vi "Leap Screen Tap Gesture.vi"() -> ()   [LabVIEW 2011, in "LVH-Leap.lvlib"]
uses:
  vi.lib/LabVIEW Hacker/Leap/LVH-Leap.lvlib
  vi.lib/LabVIEW Hacker/Leap/Public/Gestures/Screen Tap/Instance VIs/Read 1 Screen Tap Position.vi
panel:
  out "Last Screen Tap Position":cluster{"X":sgl, "Y":sgl, "Z":sgl}
  out "X Y Screen Tap Position":cluster{"X":sgl, "Z":sgl}[](graph)
  in  "Stop Button":bool
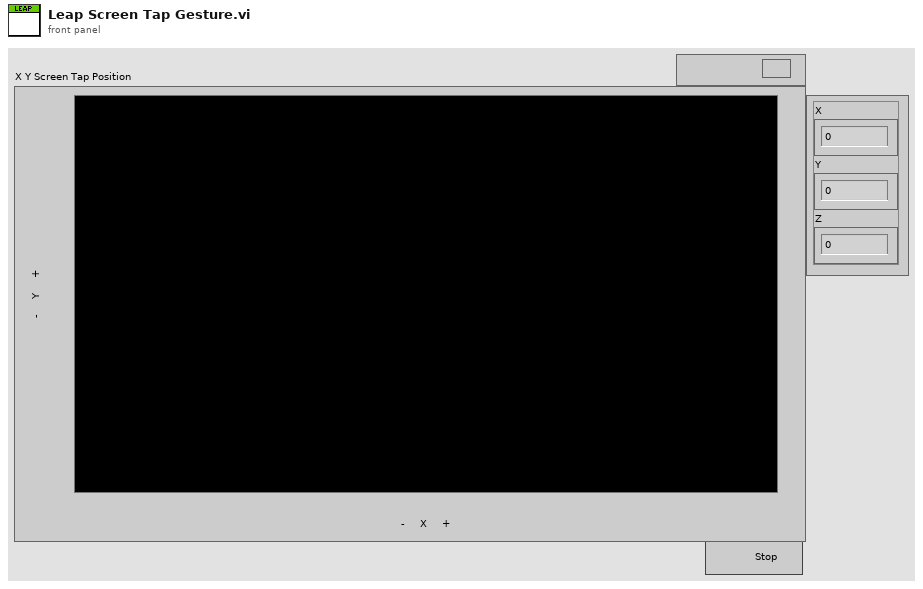
[diagram p1: front panel]
types:
  T1 = typedef "LVH-Leap.lvlib/Leap Handle.ctl" = cluster{"LeapCSharp":refnum<k24>}
  T2 = typedef "LVH-Leap.lvlib/Gesture State.ctl" = enum16{"Invalid", "Start", "Update", "Stop"}
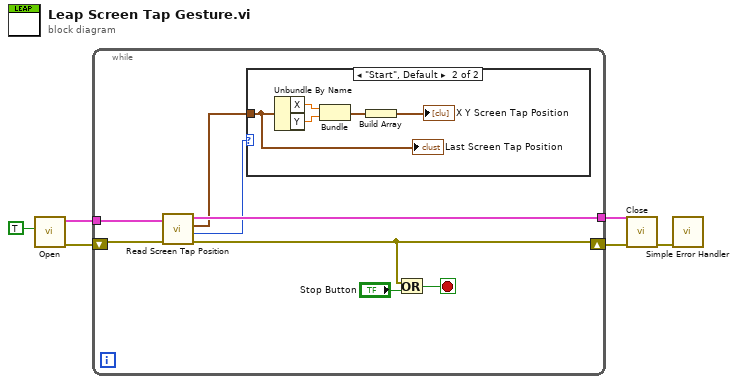
[diagram p0: block diagram]
diagram:
  n1 = call "Open.vi"("Enable Gestures? (T)"=TRUE) -> ("Error Out"=w4:errorcluster, "Leap Handle"=w6:T1)  [unwired: 9 in]
  n2 = while {
    tunnel: w6 -> [w12]
    shift-right: [w7] -> w5
    shift-left: w4 -> [w11]
    tunnel: [w10] -> w1
    stop <- w14 stop-if-true
    n3 = call-poly "Read Screen Tap Position.vi"("Error In"=w11, "Leap Handle"=w12) -> ("Error Out"=w7:errorcluster, "Screen Tap Status"=w8:T2, "Screen Tap Position"=w9:cluster{"X":sgl, "Y":sgl, "Z":sgl}, "Leap Handle"=w10:T1)  [unwired: 6 in]
    n4 = case shown="\"Start\", Default" w8 {
      tunnel: w9 -> [_ w19]
      frame "Invalid" {
      }
      frame "Start", Default {
        n5 = Unbundle By Name(w19) -> ("X"=w18:sgl, "Y"=w17:sgl)
        n6 = Bundle("X"=w18, "Y"=w17) -> (w16:cluster{"X":sgl, "Y":sgl})  [unwired: 1 in]
        n7 = Build Array(w16) -> (→"X Y Screen Tap Position":cluster{"X":sgl, "Y":sgl}[])
        "Last Screen Tap Position" <- w19
      }
    }
    n8 = Or(x=w7, y="Stop Button") -> (x .or. y?=w14:bool)
  }
  n9 = call "Close.vi"("Error In"=w5, "Leap Handle"=w1) -> ("Error Out"=w2:errorcluster)  [unwired: 9 in]
  n10 = call <vilib>:"Simple Error Handler.vi"("error in (no error)"=w2) -> ()  [unwired: 4 in, 5 out]
